vi "UImain.vi"() -> ()   [LabVIEW 2013]
uses:
  Inputmeas.ctl
  <vilib>/Statnett/LabVIEW2013 PMU Reference Library/labview-statnett-prl/PMU Recorder Light/PMU Recorder Light.lvlib
panel:
  out "Positive Sequence Voltage 1":waveform(sgl)(graph)
  out "Positive Sequence Voltage 2":waveform(sgl)(graph)
  out "Positive Sequence Current 2":waveform(sgl)(graph)
  out "Has Data":bool
  out "Input signal  fed to control algorithm":T1(graph)
  out "Error":errorcluster
  out "Control signal":T1(graph)
  out "Shared Variable Loop Period":u32
  out "SDK Read Loop Period":u32
  out "Output Values Loop period":u32
  out "SDK Read Loop":bool
  out "Sampled Values Loop":bool
  out "Main Loop Period":u32
  in  "stop":bool
  out "Positive Sequence Current 1":waveform(sgl)(graph)
  # "Synchrophasor measurements from PMU/PDC"
  # "Signals from the NI-cRIO"
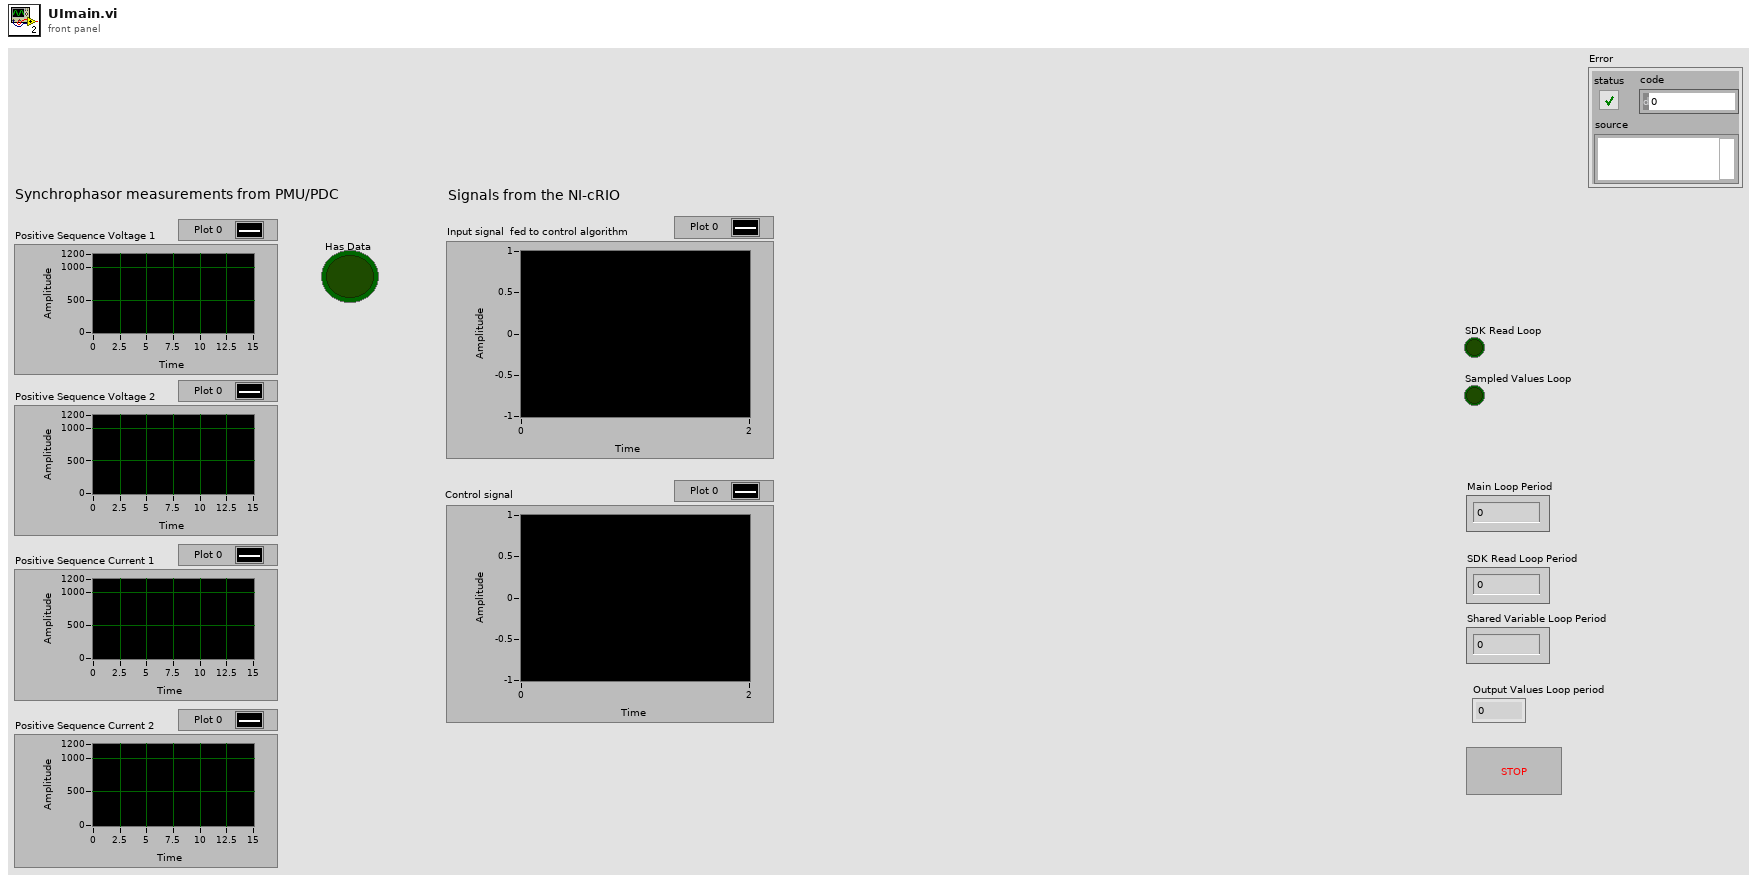
[diagram p1: front panel]
types:
  T1 = cluster{"[0]":sgl, "[1]":sgl, "[2]":sgl, "[3]":sgl, "[4]":sgl, "[5]":sgl, "[6]":sgl, "[7]":sgl, "[8]":sgl}
  T2 = cluster{"Channel 0":sgl, "Channel 1":sgl, "Channel 2":sgl, "Channel 3":sgl}
  T3 = typedef "Inputmeas.ctl" = cluster{"Time":timestamp, "Phasors":csg[]}
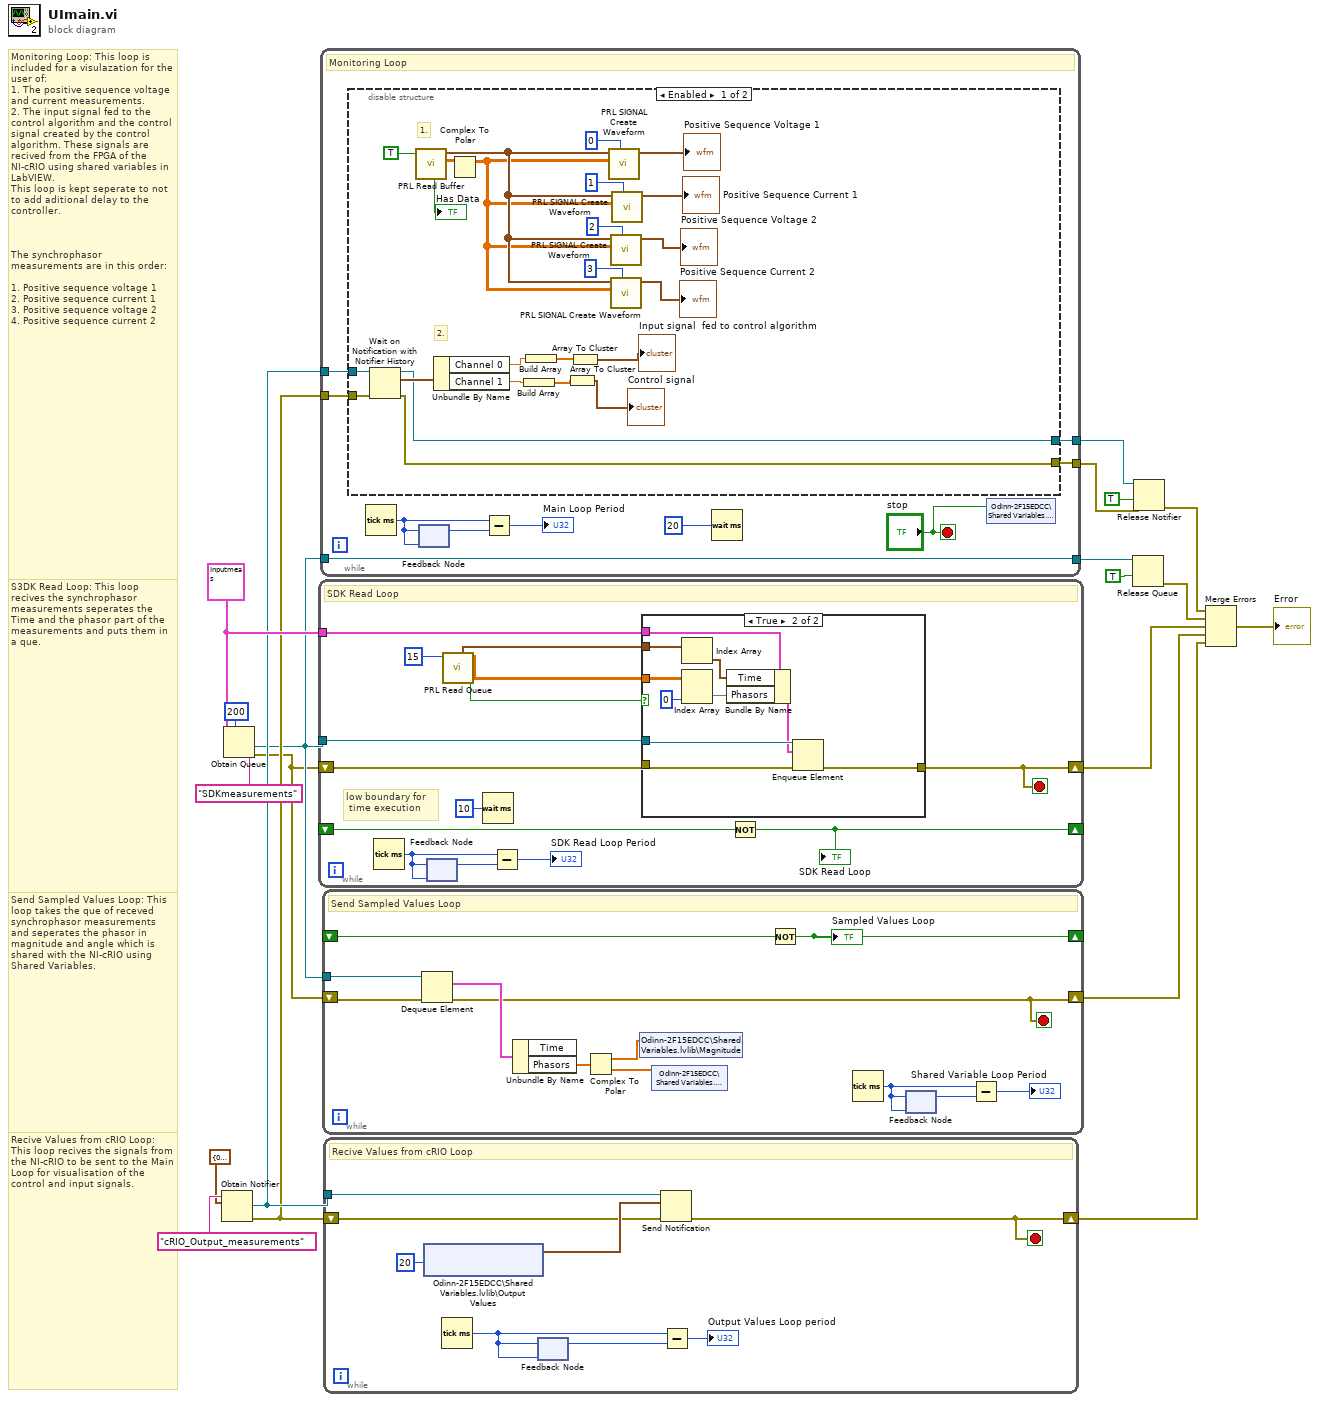
[diagram p0: block diagram]
diagram:
  w18 = T3 {"Time"=timestamp(0 s since 1904-01-01), "Phasors"=[]}
  # "Recive Values from cRIO Loop: This loop recives the signals from the NI-cRIO to be sent to the Main Loop for visualisation of the control and input signals."
  # "Send Sampled Values Loop: This loop takes the que of receved synchrophasor measurements and seperates the phasor in magnitude and angle which is shared with the NI-cRIO using Shared Variables."
  # "S3DK Read Loop: This loop recives the synchrophasor measurements seperates the Time and the phasor part of the measurements and puts them in a que."
  # "Monitoring Loop: This loop is included for a visulazation for the user of: \n1. The positive sequence voltage and current measurements.\n2. The input signal fed to the control algorithm and the control signal created by the control algorithm. These signals are recived from the FPGA of the NI-cRIO using shared variables in LabVIEW.\nThis loop is kept seperate to not to add aditional delay to the controller.\n\n\n\nThe synchrophasor measurements are in this order:\n\n1. Positive sequence voltage 1\n2. Positive sequence current 1\n3. Positive sequence voltage 2\n4. Positive sequence current 2"
  n1 = Obtain Notifier(name (unnamed)="cRIO_Output_measurements", notification data type=T2 {"Channel 0"=0.0, "Channel 1"=0.0, "Channel 2"=0.0, "Channel 3"=0.0} ("Output Values")) -> (notifier out=w14:refnum<notifier>, error out=w13:errorcluster)  [unwired: 2 in, 1 out]
  n2 = Obtain Queue(max queue size (-1, unlimited)=200, name (unnamed)="SDKmeasurements", element data type=w18) -> (queue out=w2:refnum<queue>, error out=w1:errorcluster)  [unwired: 2 in, 1 out]
  n3 = while {
    tunnel: w2 -> [w33]
    tunnel: w18 -> [w31]
    shift-right: [w28] -> w6
    shift-left: w1 -> [w32]
    shift-right: [w27] -> _
    shift-left: _ -> [w26]
    stop <- w28 stop-if-true
    # "low boundary for\n time execution"
    # "SDK Read Loop"
    n4 = Tick Count (ms)() -> (millisecond timer value=w22:u32)
    n5 = feedback #1(w22) -> (w23:u32)
    n6 = feedback-in #1(w22) -> ()
    n7 = call <vilib>:"PRL Read Queue.vi"("timeout in ms (5)"=15 ("SDK Read Timeout")) -> ("Has Data?"=w30:bool, "Phasor Values"=w25:csg[][], "Timestamp Values"=w34:timestamp[])  [unwired: 6 in, 2 out]
    n8 = Wait (ms)(milliseconds to wait=u32 10) -> ()  [unwired: 1 out]
    n9 = Subtract(x=w22, y=w23) -> (x-y=→"SDK Read Loop Period":u32)
    n10 = case shown="True" w30 {
      tunnel: w34 -> [_ w39]
      tunnel: w33 -> [_ w44]
      tunnel: w32 -> [w35 w43]
      tunnel: w31 -> [_ w42]
      tunnel: [w35 w40] -> w28
      tunnel: w25 -> [_ w36]
      frame False {
      }
      frame True {
        n11 = Index Array(array=w39) -> (element=w45:timestamp)  [unwired: 1 in]
        n12 = Index Array(array=w36, index (col)=0 ("index (row)")) -> (element=w37:csg[])  [unwired: 1 in]
        n13 = Bundle By Name(cluster=w42, "Time"=w45, "Phasors"=w37) -> (w41:T3)
        n14 = Enqueue Element(queue=w44, element=w41, error in (no error)=w43) -> (error out=w40:errorcluster)  [unwired: 1 in, 2 out]
      }
    }
    n15 = Not(x=w26) -> (.not. x?=w27:bool)
    "SDK Read Loop" <- w27
  }
  n16 = while {
    tunnel: [w52] -> w17
    tunnel: w2 -> [w52]
    tunnel: w14 -> [w50]
    tunnel: w13 -> [w49]
    tunnel: [w48] -> w12
    tunnel: [w47] -> w11
    stop <- "stop" stop-if-true
    # "Monitoring Loop"
    n17 = disable-structure shown="Enabled" {
      disable-tunnel: w50 -> [w79 _]
      disable-tunnel: w49 -> [w78 _]
      disable-tunnel: [w76 _] -> w48
      disable-tunnel: [w75 _] -> w47
      frame Enabled {
        # "2."
        # "1."
        n18 = Wait on Notification with Notifier History(0:w79, 3:w78) -> (8:w76:refnum<notifier>, 9:w77:T2, 11:w75:errorcluster)  [unwired: 2 in, 1 out]
        n19 = call <vilib>:"PRL Read Buffer .vi"("Get Full Buffer"=TRUE) -> ("Phasor Signals"=w73:csg[][], "Timestamp"=w58:timestamp[], "Has Data"=→"Has Data":bool)  [unwired: 5 in, 3 out]
        n20 = Unbundle By Name(w77) -> ("Channel 0"=w71:sgl, "Channel 1"=w70:sgl)
        n21 = Complex To Polar(r * e^(i*theta)=w73) -> (r=w57:sgl[][])  [unwired: 1 out]
        n22 = Build Array(w70) -> (w68:sgl[])
        n23 = Build Array(w71) -> (w69:sgl[])
        n24 = Array To Cluster(array=w68) -> (cluster=→"Control signal":T1)
        n25 = Array To Cluster(array=w69) -> (cluster=→"Input signal  fed to control algorithm":T1)
        n26 = call <vilib>:"PRL SIGNAL Create Waveform.vi"("Index"=0, "Analog Signals"=w57, "Timestamp"=w58) -> ("output waveform"=→"Positive Sequence Voltage 1":waveform(sgl))  [unwired: 8 in]
        n27 = call <vilib>:"PRL SIGNAL Create Waveform.vi"("Index"=2, "Analog Signals"=w57, "Timestamp"=w58) -> ("output waveform"=→"Positive Sequence Voltage 2":waveform(sgl))  [unwired: 8 in]
        n28 = call <vilib>:"PRL SIGNAL Create Waveform.vi"("Index"=3, "Analog Signals"=w57, "Timestamp"=w58) -> ("output waveform"=→"Positive Sequence Current 2":waveform(sgl))  [unwired: 8 in]
        n29 = call <vilib>:"PRL SIGNAL Create Waveform.vi"("Index"=1, "Analog Signals"=w57, "Timestamp"=w58) -> ("output waveform"=→"Positive Sequence Current 1":waveform(sgl))  [unwired: 8 in]
      }
      frame Disabled {
      }
    }
    n30 = Tick Count (ms)() -> (millisecond timer value=w54:u32)
    n31 = feedback #2(w54) -> (w55:u32)
    n32 = feedback-in #2(w54) -> ()
    n33 = Subtract(x=w54, y=w55) -> (x-y=→"Main Loop Period":u32)
    n34 = Wait (ms)(milliseconds to wait=u32 20) -> ()  [unwired: 1 out]
    n35 = shared-variable "Odinn-2F15EDCC\\Shared Variables.lvlib\\Stop"("stop") -> ()  [unwired: 1 in, 1 out]
  }
  n36 = while {
    tunnel: w2 -> [w91]
    shift-right: [w85] -> w5
    shift-left: w1 -> [w90]
    shift-right: [w87] -> _
    shift-left: _ -> [w88]
    stop <- w85 stop-if-true
    # "Send Sampled Values Loop"
    n37 = Dequeue Element(queue=w91, error in (no error)=w90) -> (element=w89:T3, error out=w85:errorcluster)  [unwired: 1 in, 2 out]
    n38 = Unbundle By Name(w89) -> ("Phasors"=w86:csg[])  [unwired: 1 out]
    n39 = Complex To Polar(r * e^(i*theta)=w86) -> (r=w81:sgl[], theta=w80:sgl[])
    n40 = shared-variable "Odinn-2F15EDCC\\Shared Variables.lvlib\\Magnitude"(w81) -> ()  [unwired: 1 in, 1 out]
    n41 = shared-variable "Odinn-2F15EDCC\\Shared Variables.lvlib\\Angle"(w80) -> ()  [unwired: 1 in, 1 out]
    n42 = Not(x=w88) -> (.not. x?=w87:bool)
    "Sampled Values Loop" <- w87
    n43 = Tick Count (ms)() -> (millisecond timer value=w83:u32)
    n44 = feedback #3(w83) -> (w84:u32)
    n45 = feedback-in #3(w83) -> ()
    n46 = Subtract(x=w83, y=w84) -> (x-y=→"Shared Variable Loop Period":u32)
  }
  n47 = while {
    tunnel: w14 -> [w93]
    shift-right: [w92] -> w4
    shift-left: w13 -> [w94]
    stop <- w92 stop-if-true
    # "Recive Values from cRIO Loop"
    n48 = shared-variable "Odinn-2F15EDCC\\Shared Variables.lvlib\\Output Values"(20 ("ms timeout (0)")) -> (w95:T2)  [unwired: 1 in, 2 out]
    n49 = Tick Count (ms)() -> (millisecond timer value=w97:u32)
    n50 = feedback #4(w97) -> (w96:u32)
    n51 = feedback-in #4(w97) -> ()
    n52 = Send Notification(notification=w95, notifier=w93, error in (no error)=w94) -> (error out=w92:errorcluster)  [unwired: 1 out]
    n53 = Subtract(x=w97, y=w96) -> (x-y=→"Output Values Loop period":u32)
  }
  n54 = Release Queue(queue=w17, force destroy? (F)=TRUE) -> (error out=w7:errorcluster)  [unwired: 1 in, 2 out]
  n55 = Release Notifier(notifier=w12, force destroy? (F)=TRUE, error in (no error)=w11) -> (error out=w8:errorcluster)  [unwired: 2 out]
  n56 = Merge Errors(w8, w7, w6, w5, w4) -> (→"Error":errorcluster)
